vi "Write Frame.vi"(8 "error in (no error)":errorcluster, 10 "Frame":waveform(cdb), 11 "Store in":refnum<class "Store.lvclass">) -> (0 "error out":errorcluster, 3 "Store out":refnum<class "Store.lvclass">)   [LabVIEW 2019, in "Store.lvclass"]
uses:
  Store.lvclass
  Store.lvclass/Store.ctl
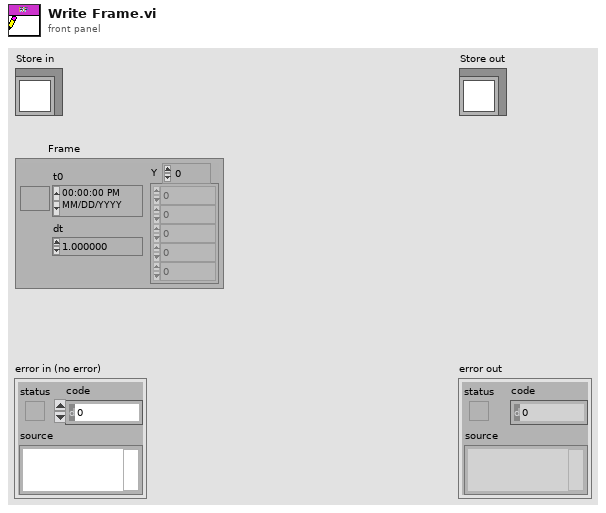
[diagram p1: front panel]
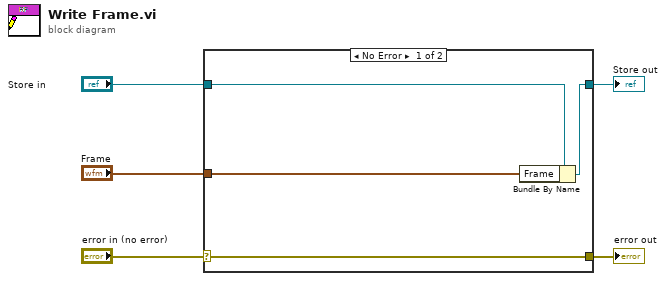
[diagram p0: block diagram]
diagram:
  n1 = case shown="No Error" "error in (no error)" {
    selector: "error in (no error)" -> [w9 w10]
    tunnel: [w9 w10] -> w4
    tunnel: [w7 w11] -> w2
    tunnel: "Store in" -> [w8 w11]
    tunnel: "Frame" -> [w6 _]
    frame No Error {
      n2 = Bundle By Name(cluster=w8, "Frame"=w6) -> (w7:refnum<class "Store.lvclass">)
    }
    frame Error {
    }
  }
  "error out" <- w4
  "Store out" <- w2
